vi "Append Numeric Table to Report.vi"(0 "report in":refnum<class "NI_Word.lvclass">, 1 "column width (1)":dbl=1.0 format="%.2f", 2 "measurement system":u16(ring)=2 caption="measurement system for column width (Default)" items=["US", "Metric", "Default"], 3 "MS Office parameters":T2, 5 "column headers":string[](array[string]), 7 "row headers":string[](array[string]), 9 "numerical data":dbl[][](array[numeric]) format="%.2f", 11 "error in (no error)":errorcluster, 12 "format string (%.3f)":string="%.3f", 13 "separate page?":bool, 14 "show grid lines":bool=TRUE) -> (4 "report out":refnum<class "NI_Word.lvclass">, 8 "range (wd) - start (xl)":T1, 10 "end (xl)":cluster{"row (xl) ":i32, "col (xl) ":i32}, 15 "error out":errorcluster)   [LabVIEW 2020, in "NI_Word.lvclass"]
doc: "Appends a 2D array to a report as a table with the given column width. You can use this polymorphic VI to append an array of strings or numbers. The data type you wire to the <B>text data</B> input determines the polymorphic instance to use."
uses:
  <vilib>/Utility/NIReport.llb/Word/NI_Word.lvclass
  <vilib>/Utility/NIReport.llb/Word/NI_Word.lvclass/NI_Word.ctl
  <vilib>/addons/_office/NI_ReportGenerationToolkit.lvlib
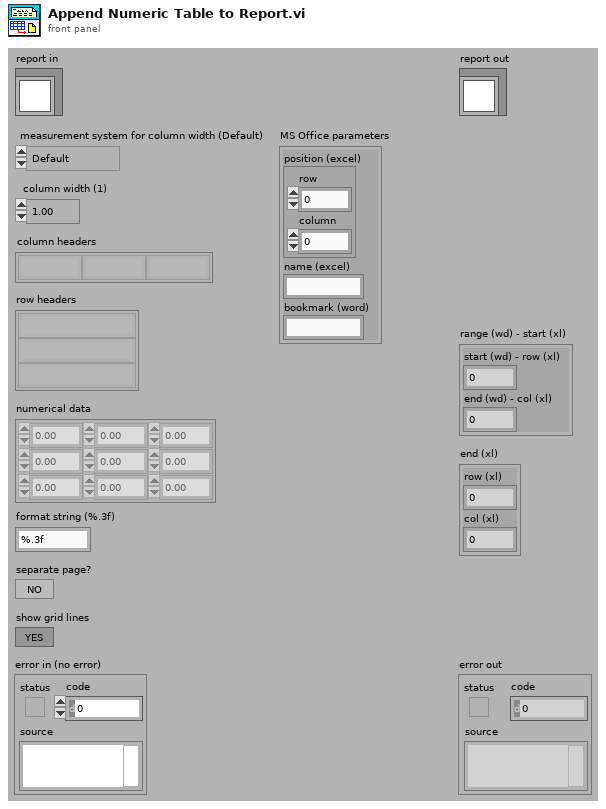
[diagram p1: front panel]
types:
  T1 = cluster{"start (wd) - row (xl) ":i32, "end (wd) - col (xl) ":i32}
  T2 = cluster{"position (excel)":cluster{"row":i32, "column":i32}, "name (excel)":string, "bookmark (word)":string}
  T3 = typedef "NI_ReportGenerationCore.lvlib/Report Data Members.ctl" = cluster{"font":T4, "from template?":bool}
  T4 = typedef "NI_ReportGenerationCore.lvlib/font.ctl" = cluster{"font name":string, "font size":dbl, "bold":u16, "italic":u16, "underline":u16, "strike through":u16, "font color":u32}
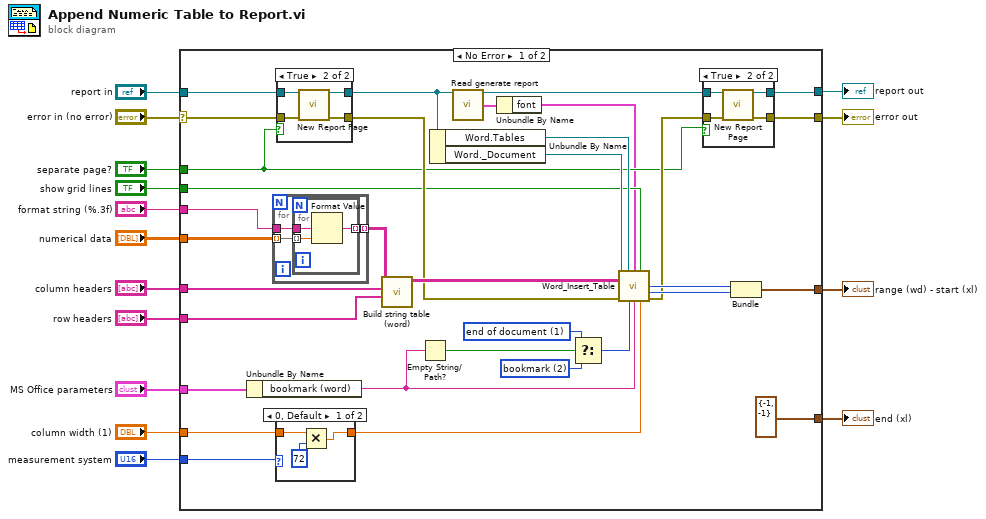
[diagram p0: block diagram]
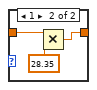
[diagram p2: hidden frame]
diagram:
  n1 = case shown="No Error" "error in (no error)" {
    selector: "error in (no error)" -> [w36 w74]
    tunnel: [w35 w74] -> w14
    tunnel: [w33 w73] -> w12
    tunnel: "report in" -> [w34 w73]
    tunnel: "show grid lines" -> [w29 _]
    tunnel: "format string (%.3f)" -> [w24 _]
    tunnel: "row headers" -> [w26 _]
    tunnel: "column headers" -> [w27 _]
    tunnel: "numerical data" -> [w25 _]
    tunnel: "column width (1)" -> [w23 _]
    tunnel: "MS Office parameters" -> [w30 _]
    tunnel: "separate page?" -> [w28 _]
    tunnel: "measurement system" -> [w22 _]
    tunnel: [w21 _] -> w2
    tunnel: [cluster{"row (xl)":i32, "col (xl)":i32} {"row (xl)"=-1, "col (xl)"=-1} ("end (xl)") _] -> w1
    frame No Error {
      w37 = u16 2 items=["begining of document", "end of document", "bookmark", "custom"] ("Insertion point")
      w38 = u16 1 items=["begining of document", "end of document", "bookmark", "custom"] ("Insertion point")
      n2 = Unbundle By Name(w30) -> ("bookmark (word)"=w42:string)
      n3 = for {
        tunnel: w25 -> [w51] mode=indexing
        tunnel: w24 -> [w50]
        tunnel: [w49] -> w40 mode=indexing
        n4 = for {
          tunnel: w51 -> [w54] mode=indexing
          tunnel: w50 -> [w53]
          tunnel: [w52] -> w49 mode=indexing
          n5 = Format Value(format string=w53, value (0)=w54) -> (output string=w52:string)  [unwired: 1 out]
        }
      }
      n6 = case shown="0, Default" w22 {
        tunnel: w23 -> [w57 w59]
        tunnel: [w56 w58] -> w41
        frame 0, Default {
          n7 = Multiply(x=w57, y=72) -> (x*y=w56:dbl)
        }
        frame 1 {
          n8 = Multiply(x=w59, y=28.35) -> (x*y=w58:dbl)
        }
      }
      n9 = case shown="True" w28 {
        tunnel: w34 -> [w68 w72]
        tunnel: w36 -> [w67 w71]
        tunnel: [w68 w70] -> w19
        tunnel: [w67 w69] -> w31
        frame False {
        }
        frame True {
          n10 = call-dynamic "New Report Page.vi"("report in"=w72, "error in (no error)"=w71) -> ("report out"=w70:refnum<class "NI_Word.lvclass">, "error out"=w69:errorcluster)  [unwired: 12 in]
        }
      }
      n11 = call <vilib>:"Build string table (word).vi"("row headers"=w26, "column headers"=w27, "text data"=w40) -> ("output table"=w45:string[][])  [unwired: 1 in, 7 out]
      n12 = Empty String/Path?(string/path=w42) -> (empty?=w39:bool)
      n13 = Unbundle By Name(w19) -> ("Word.Tables"=w46:refnum<k7>, "Word._Document"=w44:refnum<k7>)
      n14 = call-dynamic "Read generate report.vi"("report in"=w19) -> ("report out"=w18:refnum<class "NI_Word.lvclass">, "generate report"=w17:T3)  [unwired: 12 in, 1 out]
      n15 = Unbundle By Name(w17) -> ("font"=w16:T4)
      n16 = Select(t=w38, s=w39, f=w37) -> (s? t:f=w43:u16)
      n17 = call <vilib>:"Word_Insert_Table.vi"("Document"=w44, "Tables"=w46, "font"=w16, "show grid lines"=w29, "Table data"=w45, "error in (no error)"=w31, "Insertion point"=w43, "Bookmark name"=w42, "column width (1)"=w41) -> ("Start out"=w47:i32, "End out"=w48:i32, "error out"=w32:errorcluster)  [unwired: 2 in, 2 out]
      n18 = case shown="True" w28 {
        tunnel: [w62 w66] -> w33
        tunnel: [w61 w65] -> w35
        tunnel: w32 -> [w61 w64]
        tunnel: w18 -> [w62 w63]
        frame False {
        }
        frame True {
          n19 = call-dynamic "New Report Page.vi"("report in"=w63, "error in (no error)"=w64) -> ("report out"=w66:refnum<class "NI_Word.lvclass">, "error out"=w65:errorcluster)  [unwired: 12 in]
        }
      }
      n20 = Bundle("Start out"=w47, "End out"=w48) -> (w21:cluster{"Start out":i32, "End out":i32})  [unwired: 1 out]
    }
    frame Error {
    }
  }
  "error out" <- w14
  "report out" <- w12
  "end (xl)" <- w1
  "range (wd) - start (xl)" <- w2
